vi "Check if Click in Graph Legend.vi"(8 "error in (no error)":errorcluster, 10 "Mouse Coords":T1, 11 "WaveformGraph":refnum<vi>) -> (0 "error out":errorcluster, 2 "click in legend?":bool)   [LabVIEW 2022 SP3, in "UI Helpers.lvlib"]
uses:
  UI Helpers.lvlib
  <vilib>/Utility/miscctls.llb/LVPoint32TypeDef.ctl
  <vilib>/Utility/miscctls.llb/LVPointTypeDef.ctl
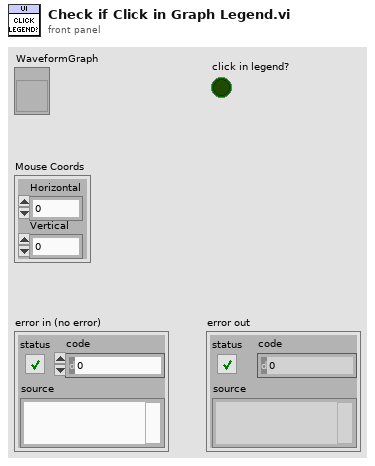
[diagram p1: front panel]
types:
  T1 = typedef "LVPoint32TypeDef.ctl" = cluster{"Horizontal":i32, "Vertical":i32}
  T2 = typedef "LVPointTypeDef.ctl" = cluster{"Horizontal":i16, "Vertical":i16}
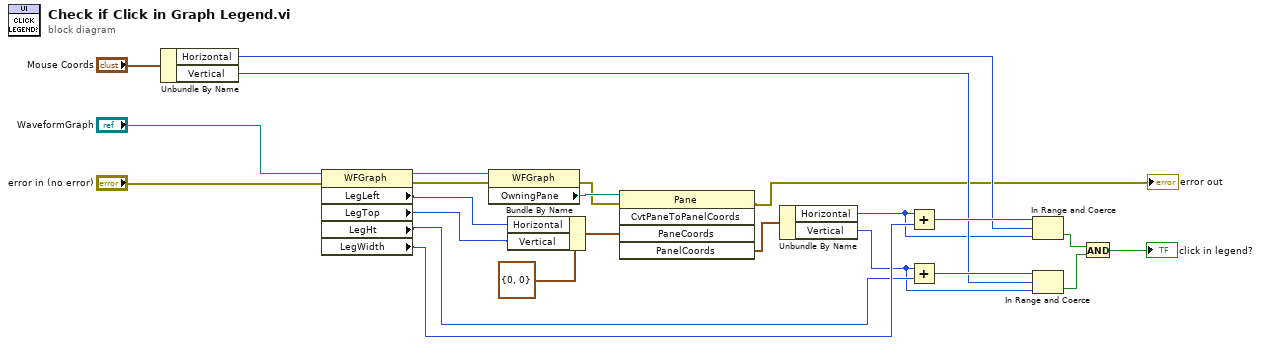
[diagram p0: block diagram]
diagram:
  n1 = Unbundle By Name("Mouse Coords") -> ("Horizontal"=w19:i32, "Vertical"=w18:i32)
  n2 = property class="WFGraph"(reference="WaveformGraph", error in="error in (no error)") -> (reference out=w14:refnum<vi>, error out=w13:errorcluster, "LegLeft"=w8:i32, "LegTop"=w7:i32, "LegHt"=w3:u32, "LegWidth"=w4:u32)
  n3 = property class="WFGraph"(reference=w14, error in=w13) -> (error out=w11:errorcluster, "OwningPane"=w12:refnum<vi>)  [unwired: 1 out]
  n4 = Bundle By Name(cluster=T2 {"Horizontal"=0, "Vertical"=0} ("Pane Coordinates"), "Horizontal"=w8, "Vertical"=w7) -> (w9:T2)
  n5 = invoke class="Pane" method="CvtPaneToPanelCoords"(reference=w12, error in=w11, "PaneCoords"=w9) -> (error out=→"error out":errorcluster, "PanelCoords"=w5:T2)  [unwired: 2 in, 3 out]
  n6 = Unbundle By Name(w5) -> ("Horizontal"=w2:i16, "Vertical"=w1:i16)
  n7 = Add(x=w2, y=w4) -> (x+y=w22:u32)
  n8 = Add(x=w1, y=w3) -> (x+y=w21:u32)
  n9 = In Range and Coerce(upper limit=w22, x=w19, lower limit=w2) -> (In Range?=w17:bool)  [unwired: 1 out]
  n10 = In Range and Coerce(upper limit=w21, x=w18, lower limit=w1) -> (In Range?=w16:bool)  [unwired: 1 out]
  n11 = And(x=w17, y=w16) -> (x .and. y?=→"click in legend?":bool)
